vi "Test Set Subpanels-- Config-- Maui 2.0 Default.vi"(8 "error in":errorcluster) -> (0 "error out":errorcluster)   [LabVIEW 2019]
uses:
  <vilib>/JKI/JKI SMO/SMO/SMO.lvclass
  Maui 2.0/Maui 2.0.lvclass
  <vilib>/Utility/config.llb/NI_LVConfig.lvlib
  <vilib>/addons/_JKI Toolkits/Caraya/classes/Test/Test.lvclass
  <vilib>/addons/_JKI Toolkits/Caraya/classes/Assert/Assert.lvclass
  <vilib>/addons/_JKI Toolkits/Caraya/classes/Assert/Assert True.vi
  C:/Program Files (x86)/National Instruments/LabVIEW 2020/vi.lib/JKI/JKI SMO/SMO/SMO.lvclass
  Maui 2.0/Typedefs/Maui 2.0/Maui 2.0 Configuration.ctl
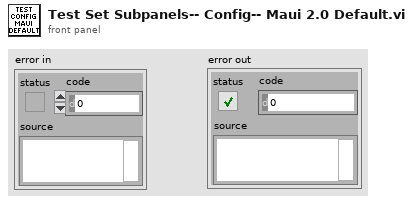
[diagram p1: front panel]
types:
  T1 = typedef "Maui 2.0.lvclass/Maui 2.0 Configuration.ctl" = cluster{"Paths":path[]}
  T2 = typedef "NI_LVConfig.lvlib/Config Data RefNum.ctl" = refnum<k1>
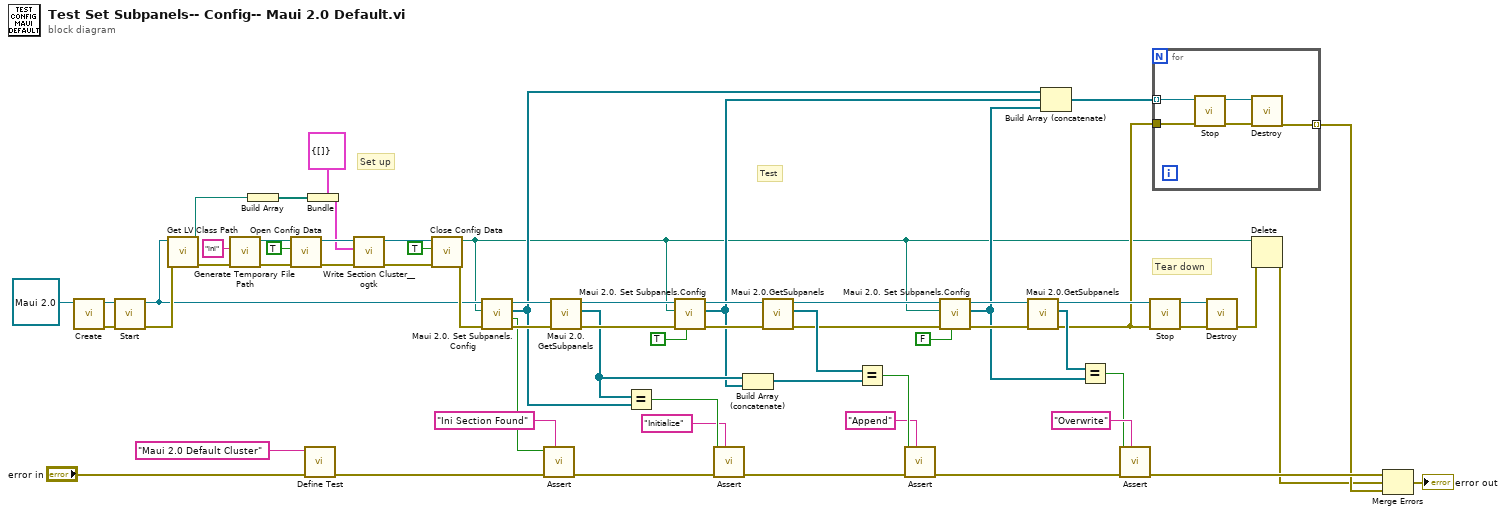
[diagram p0: block diagram]
diagram:
  # "Tear down"
  # "Test"
  # "Set up"
  n1 = call <vilib>:"Create.vi"("SMO"=refnum<class "Maui 2.0.lvclass"> refnum ("Maui 2.0.lvclass")) -> ("error out"=w64:errorcluster, "SMO out"=w54:refnum<class "Maui 2.0.lvclass">)  [unwired: 8 in, 1 out]
  n2 = call <vilib>:"Start.vi"("error in (no error)"=w64, "SMO"=w54) -> ("error out"=w62:errorcluster, "SMO out"=w47:refnum<class "Maui 2.0.lvclass">)  [unwired: 8 in]
  n3 = call <vilib>:"Get LV Class Path.vi"("error in (no error)"=w62, "object"=w47) -> ("error out"=w8:errorcluster, "class path"=w6:path)  [unwired: 8 in]
  n4 = call <vilib>:"Generate Temporary File Path.vi"("error in (no error)"=w8, "Temporary File Extension (tmp)"="ini") -> ("error out"=w7:errorcluster, "Unique Temporary File Path"=w4:path)  [unwired: 8 in]
  n5 = Build Array(w6) -> (w50:path[])
  n6 = call <vilib>:"Open Config Data.vi"("error in (no error)"=w7, "create file if necessary (T)"=TRUE, "configuration file path"=w4) -> ("error out"=w61:errorcluster, "refnum"=w51:T2)  [unwired: 6 in, 1 out]
  n7 = call <vilib>:"Define Test.vi"("error in (no error)"="error in", "Label (VI Title)"="Maui 2.0 Default Cluster") -> ("error out"=w57:errorcluster)  [unwired: 9 in]
  n8 = Bundle(cluster=T1 {"Paths"=[]} ("Subpanels"), "Paths"=w50) -> (w2:T1)
  n9 = call "Write Section Cluster__ogtk.vi"("error in (no error)"=w61, "Section Formatted Cluster"=w2, "refnum"=w51) -> ("error out"=w60:errorcluster, "dup refnum"=w49:T2)  [unwired: 7 in]
  n10 = call <vilib>:"Close Config Data.vi"("error in (no error)"=w60, "write file if changed (T)"=TRUE, "refnum"=w49) -> ("error out"=w56:errorcluster, "file path"=w10:path)  [unwired: 7 in]
  n11 = call-dynamic "Maui 2.0. Set Subpanels.Config.vi"("error in"=w56, "Path"=w10, "Maui 2.0 in"=w47) -> ("error out"=w59:errorcluster, "Found?"=w20:bool, "Subpanels"=w17:refnum<class "SMO.lvclass">[], "Maui 2.0 out"=w46:refnum<class "Maui 2.0.lvclass">)  [unwired: 5 in]
  n12 = call-poly <vilib>:"Assert.vi"("Label"="Ini Section Found", "error in (no error)"=w57, "True?"=w20) -> ("error out"=w58:errorcluster)  [unwired: 8 in]
  n13 = call "Maui 2.0.GetSubpanels.vi"("error in (no error)"=w59, "Maui 2.0"=w46) -> ("error out"=w42:errorcluster, "Subpanels"=w31:refnum<class "SMO.lvclass">[], "Maui 2.0 out"=w36:refnum<class "Maui 2.0.lvclass">)  [unwired: 7 in]
  n14 = Equal?(x=w31, y=w17) -> (x = y?=w14:bool)
  n15 = call-dynamic "Maui 2.0. Set Subpanels.Config.vi"("Append (F)"=TRUE, "error in"=w42, "Path"=w10, "Maui 2.0 in"=w36) -> ("error out"=w43:errorcluster, "Subpanels"=w18:refnum<class "SMO.lvclass">[], "Maui 2.0 out"=w44:refnum<class "Maui 2.0.lvclass">)  [unwired: 4 in, 1 out]
  n16 = call-poly <vilib>:"Assert.vi"("Label"="Initialize", "error in (no error)"=w58, "True?"=w14) -> ("error out"=w39:errorcluster)  [unwired: 8 in]
  n17 = Build Array (concatenate)(w31, w18) -> (w35:refnum<class "SMO.lvclass">[])
  n18 = call "Maui 2.0.GetSubpanels.vi"("error in (no error)"=w43, "Maui 2.0"=w44) -> ("error out"=w25:errorcluster, "Subpanels"=w40:refnum<class "SMO.lvclass">[], "Maui 2.0 out"=w26:refnum<class "Maui 2.0.lvclass">)  [unwired: 7 in]
  n19 = Equal?(x=w40, y=w35) -> (x = y?=w38:bool)
  n20 = call-poly <vilib>:"Assert.vi"("Label"="Append", "error in (no error)"=w39, "True?"=w38) -> ("error out"=w30:errorcluster)  [unwired: 8 in]
  n21 = call-dynamic "Maui 2.0. Set Subpanels.Config.vi"("Append (F)"=FALSE, "error in"=w25, "Path"=w10, "Maui 2.0 in"=w26) -> ("error out"=w28:errorcluster, "Subpanels"=w19:refnum<class "SMO.lvclass">[], "Maui 2.0 out"=w27:refnum<class "Maui 2.0.lvclass">)  [unwired: 4 in, 1 out]
  n22 = call "Maui 2.0.GetSubpanels.vi"("error in (no error)"=w28, "Maui 2.0"=w27) -> ("error out"=w11:errorcluster, "Subpanels"=w23:refnum<class "SMO.lvclass">[], "Maui 2.0 out"=w24:refnum<class "Maui 2.0.lvclass">)  [unwired: 7 in]
  n23 = Build Array (concatenate)(w17, w18, w19) -> (w16:refnum<class "SMO.lvclass">[])
  n24 = Equal?(x=w23, y=w19) -> (x = y?=w12:bool)
  n25 = call-poly <vilib>:"Assert.vi"("Label"="Overwrite", "error in (no error)"=w30, "True?"=w12) -> ("error out"=w29:errorcluster)  [unwired: 8 in]
  n26 = call <vilib>:"Stop.vi"("error in (no error)"=w11, "SMO"=w24) -> ("error out"=w63:errorcluster, "SMO out"=w53:refnum<class "Maui 2.0.lvclass">)  [unwired: 8 in]
  n27 = for {
    tunnel: w16 -> [w67] mode=indexing
    tunnel: [w66] -> w15 mode=indexing
    tunnel: w11 -> [w65]
    n28 = call <vilib>:"Stop.vi"("error in (no error)"=w65, "SMO"=w67) -> ("error out"=w68:errorcluster, "SMO out"=w69:refnum<class "SMO.lvclass">)  [unwired: 8 in]
    n29 = call <vilib>:"Destroy.vi"("error in (no error)"=w68, "SMO"=w69) -> ("error out"=w66:errorcluster)  [unwired: 9 in]
  }
  n30 = call <vilib>:"Destroy.vi"("error in (no error)"=w63, "SMO"=w53) -> ("error out"=w9:errorcluster)  [unwired: 9 in]
  n31 = Delete(path (use dialog)=w10, error in=w9) -> (error out=w3:errorcluster)  [unwired: 3 in, 2 out]
  n32 = Merge Errors(w29, w3, w15) -> (→"error out":errorcluster)
